vi "check log file size.vi"() -> ()   [LabVIEW 2013]
uses:
  ctl/q_data.ctl
  ctl/UI_cmd-ctl.ctl
  Global.vi
panel:
  out "데이터":T1
  out "x-y":i64
  out "error out":errorcluster
  in  "error in":errorcluster
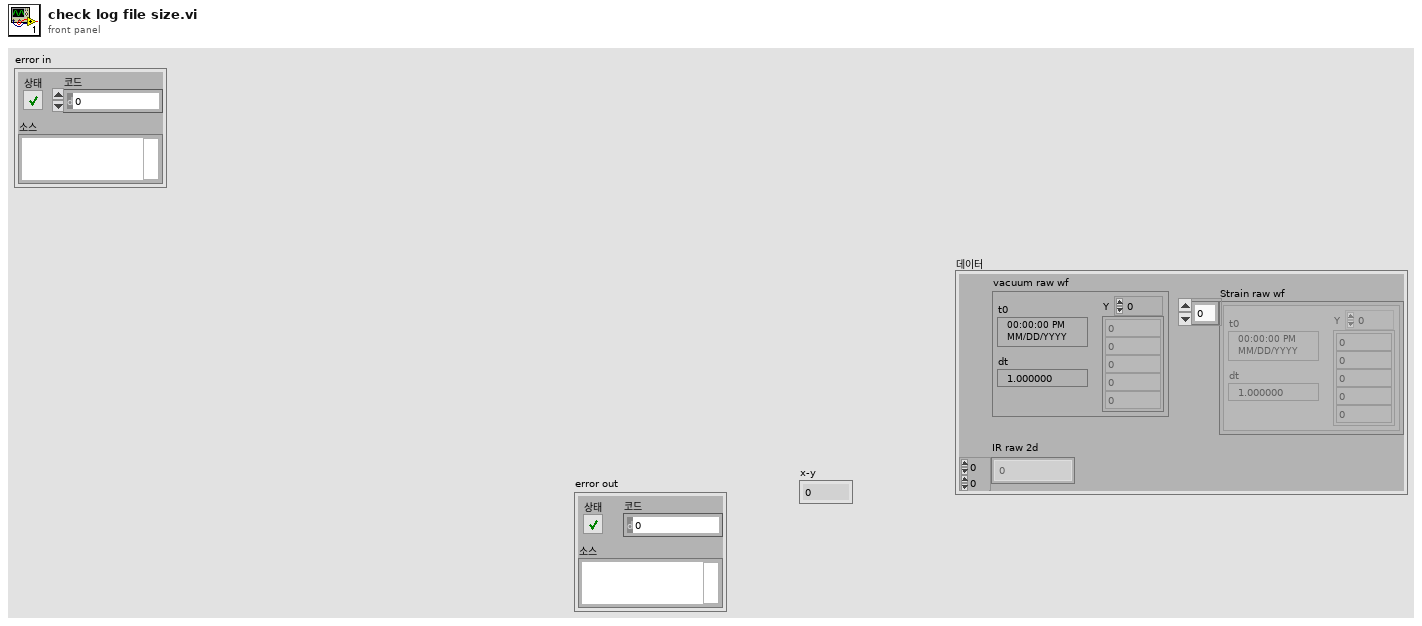
[diagram p1: front panel]
types:
  T1 = typedef "q_data.ctl" = cluster{"Strain raw wf":waveform(dbl)[], "vacuum raw wf":waveform(dbl), "IR raw 2d":i16[][]}
  T2 = typedef "UI_cmd-ctl.ctl" = enum16{"default", "create", "read"}
  T3 = cluster{"simulation file path":path, "simulation speed":u32}
  T4 = typedef "UI_ctl2.ctl" = cluster{"simulation status":refnum<vi>}
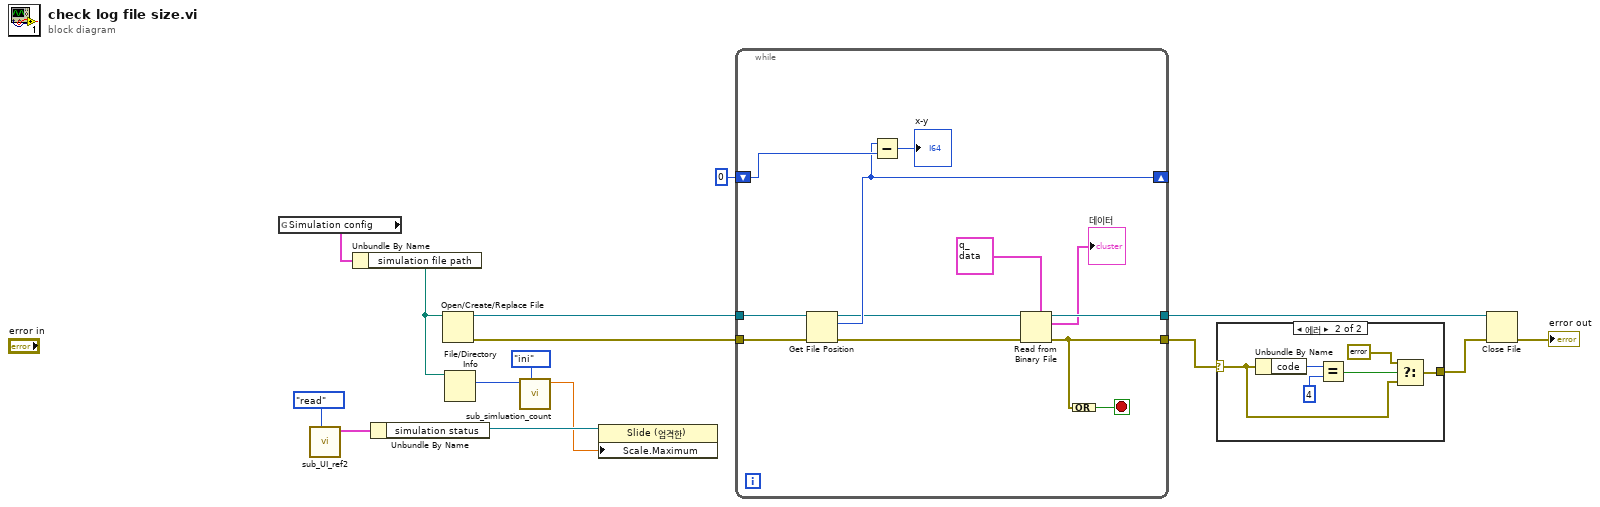
[diagram p0: block diagram]
diagram:
  n1 = global read "Global.vi" "Simulation config"() -> (w9:T3)
  n2 = call "sub_UI_ref2.vi"("cmd"=UI_cmd-ctl."read") -> ("UI ctl2 out"=w6:T4)  [unwired: 10 in]
  n3 = Unbundle By Name(w9) -> ("simulation file path"=w8:path)
  n4 = Unbundle By Name(w6) -> ("simulation status"=w5:refnum<vi>)
  n5 = Open/Create/Replace File(file path (use dialog)=w8) -> (refnum out=w12:refnum<file>, error out=w14:errorcluster)  [unwired: 5 in, 1 out]
  n6 = File/Directory Info(path=w8) -> (size=w4:i64)  [unwired: 1 in, 6 out]
  n7 = call "sub_simluation_count.vi"("cmd"=enum16{"ini", "count"}."ini", "data"=w4) -> ("max"=w2:dbl)  [unwired: 8 in, 1 out]
  n8 = property class="Slide (엄격한)"(reference=w5, "Scale.Maximum"=w2) -> ()  [unwired: 1 in, 2 out]
  n9 = while {
    tunnel: w14 -> [w19]
    tunnel: [w26] -> w11
    tunnel: [w25] -> w13
    tunnel: w12 -> [w21]
    shift-right: [w23] -> _
    shift-left: i64 0 ("offset (in bytes)") -> [w24]
    stop <- w27 stop-if-true
    n10 = Get File Position(4:w19, 7:w21) -> (0:w18:errorcluster, 2:w23:i64, 3:w20:refnum<file>)
    n11 = Subtract(x=w23, y=w24) -> (x-y=→"x-y":i64)
    n12 = Read from Binary File(5:T1 {"Strain raw wf"=[{"t0"=timestamp(0 s since 1904-01-01), "dt"=0.00062, "Y"=[]}], "vacuum raw wf"={"t0"=timestamp(0 s since 1904-01-01), "dt"=0.00062, "Y"=[]}, "IR raw 2d"=[]} ("Q_data"), 8:w18, 11:w20) -> (0:w26:errorcluster, 2:→"데이터":T1, 3:w25:refnum<file>)  [unwired: 3 in, 1 out]
    n13 = Compound Arithmetic op=OR(w26) -> (w27:bool)
  }
  n14 = case shown="에러" w11 {
    selector: w11 -> [w28 w29]
    tunnel: [w28 w30] -> w10
    frame No Error {
    }
    frame Error {
      n15 = Unbundle By Name(w29) -> ("code"=w34:i32)
      n16 = Equal?(x=w34, y=4) -> (x = y?=w32:bool)
      n17 = Select(t=errorcluster {"status"=FALSE, "code"=0, "source"=""} ("error IO"), s=w32, f=w29) -> (s? t:f=w30:errorcluster)
    }
  }
  n18 = Close File(refnum=w13, error in=w10) -> (error out=→"error out":errorcluster)  [unwired: 1 out]
